vi "Real_Time_Main_Final_Digital.vi"() -> ()   [LabVIEW 2024]
uses:
  <vilib>/Platform/TimedLoop/XDataNode/timing_clust.ctl
  <vilib>/Platform/TimedLoop/XDataNode/nitl_modes.ctl
  <vilib>/Platform/TimedLoop/XDataNode/wakeup.ctl
  <instrlib>/niScope/Controls/niScope vertical coupling.ctl
  <instrlib>/niScope/Configure/Trigger/niScope Configure Trigger Digital.vi
  <instrlib>/niScope/Acquire/Fetch/niScope Fetch WDT.vi
  <vilib>/platform/TimedLoop/XDataNode/XDataNode.xnode
  <instrlib>/niScope/Controls/niScope trigger source digital.ctl
  <vilib>/Platform/TimedLoop/XDataNode/XDNodeRunTimeDep.lvlib
panel:
  out "output waveform":waveform(dbl)(graph)
  in  "trigger source":T1="VAL_RTSI_0"
  out "error out":errorcluster
  in  "Fetch:Fetch Relative To":i32(ring)=482 items=["Start"=482, "Trigger"=483, "Pretrigger"=477, "Now"=481, "Read Pointer"=388]
  out "# of Chunks Fetched":i32
  out "# of Points Fetched":i32
  out "Horizontal:Actual Sample Rate":dbl
  in  "channels":string="0"
  in  "stop":bool
  in  "Resource Name":refnum<k15>="Dev1" caption="Resource Name(s)"
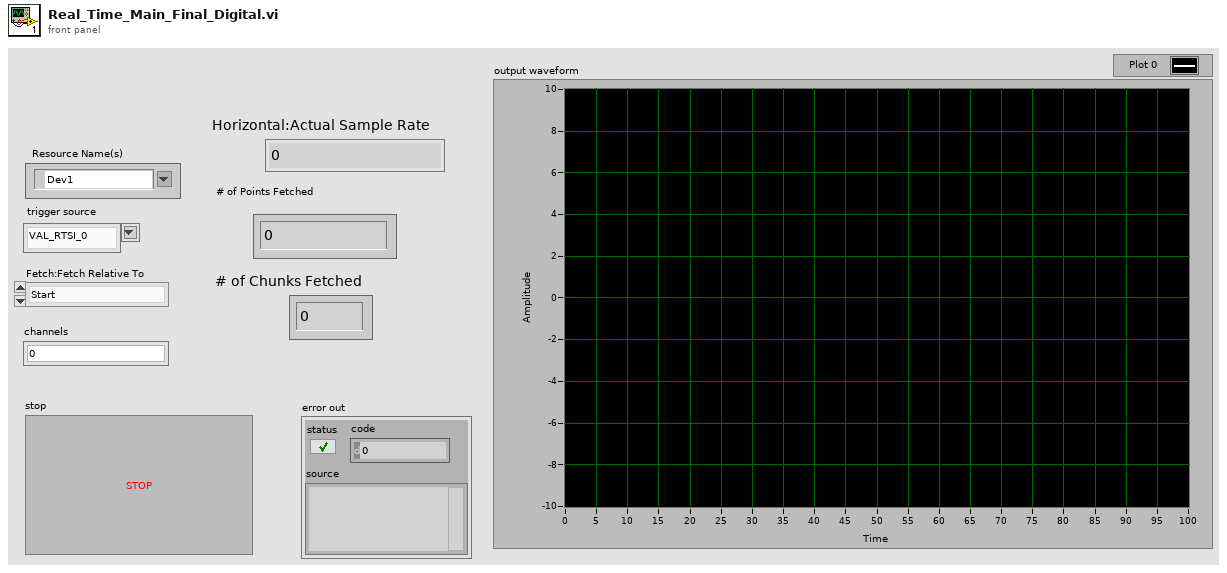
[diagram p1: front panel]
types:
  T1 = typedef "niScope trigger source digital.ctl" = string
  T2 = typedef "XDNodeRunTimeDep.lvlib/timing_clust.ctl" = cluster{"Expected End [f-1]":u64, "Actual End [f-1]":u64, "Finished Late? [f-1]":bool, "Expected End [i-1]":u64, "Actual End [i-1]":u64, "Finished Late? [i-1]":bool, "Expected Start [i]":u64, "Actual Start [i]":u64, "Expected Start [f]":u64, "Actual Start [f]":u64, "Source Name":string, "Structure Name":string, "Period":i64, "Deadline":i64, "Offset":i64, "Start":i64, "Priority":i32, "Timeout":i32, "Mode":T3, "Wakeup Reason":T4, "Error":errorcluster, "Source Type":string, "Secondary Source Type":string, "Global End Time":u64, "Global Start Time":u64, "Frame Duration":u64, "Iteration Duration":u64, "Assigned CPU":i32, "I/O Scan Engine Mode":u32}
  T3 = typedef "XDNodeRunTimeDep.lvlib/nitl_modes.ctl" = enum32{"No Change", "Process missed periods, maintain original phase", "Discard missed periods, maintain original phase", "Process missed periods, ignore original phase", "Discard missed periods, ignore original phase"}
  T4 = typedef "XDNodeRunTimeDep.lvlib/wakeup.ctl" = enum32{"Normal", "Aborted", "Asynchronous wakeup", "Timing source error", "Timed loop error", "Timeout"}
  T5 = typedef "niScope vertical coupling.ctl" = i32
  T6 = cluster{"actualSamples":i32, "absoluteInitialX":dbl, "relativeInitialX":dbl, "xIncrement":dbl, "offset":dbl, "gain":dbl, "reserved1":dbl, "reserved2":dbl}
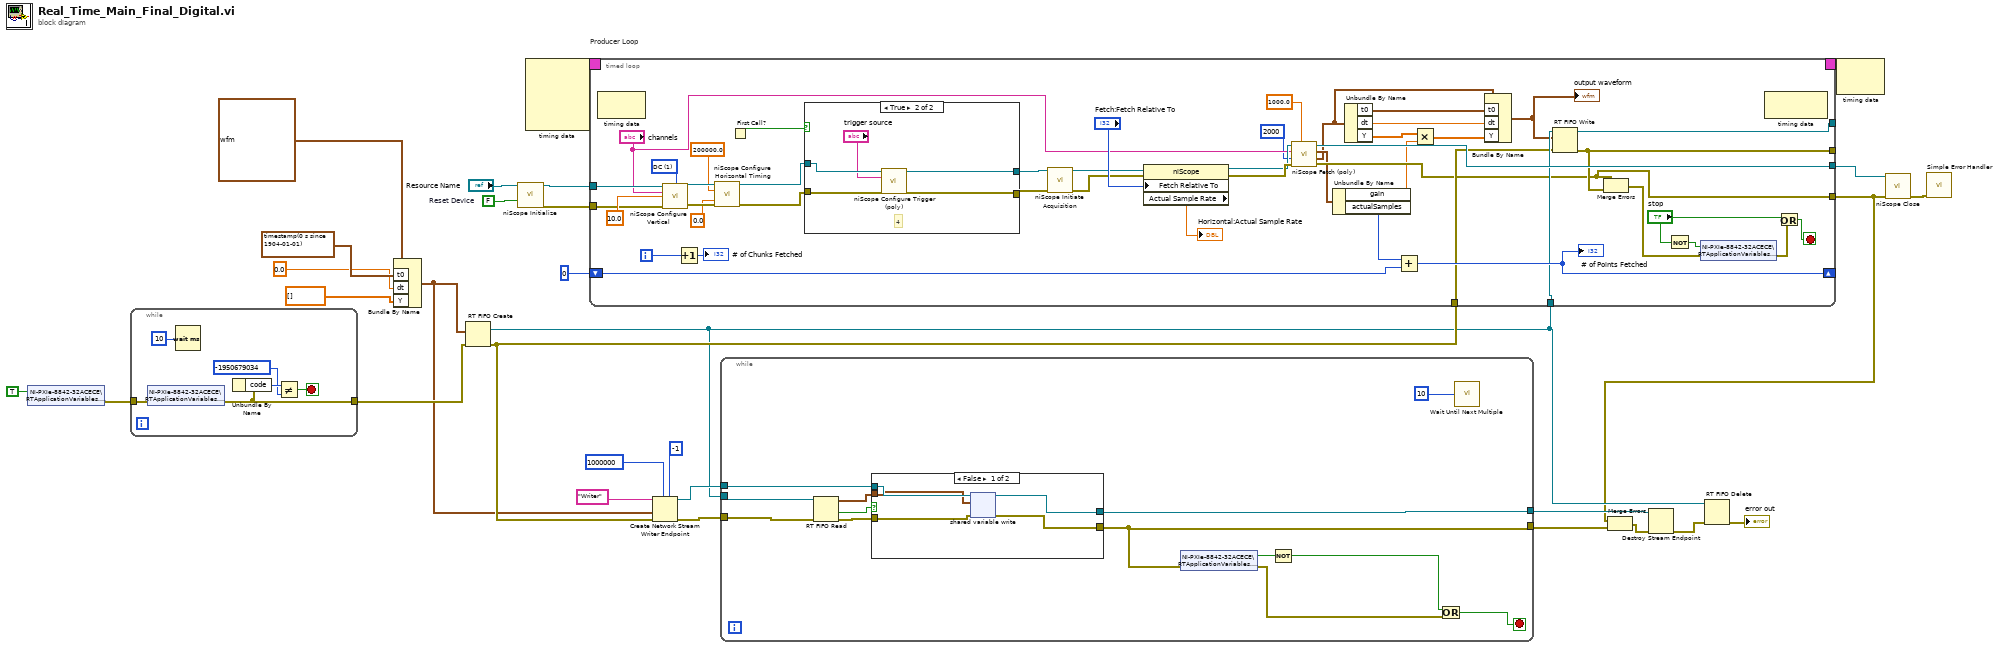
[diagram p0: block diagram]
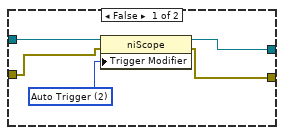
[diagram p3: hidden frame]
diagram:
  w28 = FALSE  # Reset Device
  n1 = shared-variable "NI-PXIe-8842-32ACECE\\RTApplicationVariables.lvlib\\Running?"(TRUE) -> (error out=w9:errorcluster)  [unwired: 1 in]
  n2 = while {
    tunnel: w9 -> [w36]
    tunnel: [w31] -> w8
    stop <- w33 stop-if-true
    n3 = shared-variable "NI-PXIe-8842-32ACECE\\RTApplicationVariables.lvlib\\Running?"(error in=w36) -> (error out=w31:errorcluster)  [unwired: 1 out]
    n4 = Wait (ms)(milliseconds to wait=u32 10) -> ()  [unwired: 1 out]
    n5 = Unbundle By Name(w31) -> ("code"=w35:i32)
    n6 = Not Equal?(x=w35, y=-1950679034) -> (x != y?=w33:bool)
  }
  n7 = Bundle By Name(cluster=waveform(dbl) {"t0"=timestamp(0 s since 1904-01-01), "dt"=1.0, "Y"=[]} ("waveform"), "t0"=timestamp(0 s since 1904-01-01), "dt"=0.0, "Y"=dbl[] []) -> (w3:waveform(dbl))
  n8 = RT FIFO Create(1:w3, 3:w8) -> (8:w11:refnum<k33>, 11:w21:errorcluster)  [unwired: 6 in, 1 out]
  n9 = call <instrlib>:"niScope Initialize.vi"("resource name"="Resource Name", "reset device"=w28) -> ("instrument handle"=w24:refnum<k15>, "error out"=w1:errorcluster)  [unwired: 12 in]
  n10 = node-c288() -> (w30:T2)  [unwired: 4 in]
  n11 = timed-loop "Producer Loop" {
    timing: w30 -> [_]
    timing-out: [_] -> w29
    tunnel: [w71] -> w26
    shift-right: [w69] -> _
    shift-left: 0 -> [w70]
    tunnel: w24 -> [w60]
    tunnel: w11 -> [w56]
    tunnel: w21 -> [w55]
    tunnel: [w54] -> _
    tunnel: [w53] -> _
    tunnel: [w47] -> w7
    tunnel: w1 -> [w37]
    i -> [w68]
    stop <- w50 stop-if-true
    w64 = T5 1 items=["AC", "DC", "Ground"] ("vertical coupling")
    n12 = node-c288() -> ()  [unwired: 1 in, 1 out]
    n13 = call <instrlib>:"niScope Configure Vertical.vi"("instrument handle"=w60, "vertical coupling"=w64, "channels"="channels", "vertical range"=10.0, "error in"=w37) -> ("instrument handle out"=w67:refnum<k15>, "error out"=w61:errorcluster)  [unwired: 9 in]
    n14 = Increment(x=w68) -> (x+1=→"# of Chunks Fetched":i32)
    n15 = call <instrlib>:"niScope Configure Horizontal Timing.vi"("instrument handle"=w67, "min sample rate"=200000.0, "reference position"=0.0, "error in"=w61) -> ("instrument handle out"=w62:refnum<k15>, "error out"=w63:errorcluster)  [unwired: 10 in]
    n16 = First Call?() -> (First Call?: T/F=w81:bool)
    n17 = case shown="True" w81 {
      tunnel: [w86 w92] -> w82
      tunnel: [w87 w91] -> w73
      tunnel: w63 -> [w84 w90]
      tunnel: w62 -> [w83 w89]
      frame False {
        w85 = 2 items=["None"=1, "Auto Trigger"=2] ("Triggering:Trigger Modifier")
        n18 = property class="niScope"(reference=w83, error in=w84, "Trigger Modifier"=w85) -> (reference out=w87:refnum<k15>, error out=w86:errorcluster)
      }
      frame True {
        # "4"
        n19 = call-poly <instrlib>:"niScope Configure Trigger (poly).vi"("instrument handle"=w89, "trigger source"="trigger source", "error in"=w90) -> ("instrument handle out"=w91:refnum<k15>, "error out"=w92:errorcluster)  [unwired: 11 in]
      }
    }
    n20 = call <instrlib>:"niScope Initiate Acquisition.vi"("instrument handle"=w73, "error in"=w82) -> ("instrument handle out"=w74:refnum<k15>, "error out"=w79:errorcluster)  [unwired: 12 in]
    n21 = property class="niScope"(reference=w74, error in=w79, "Fetch Relative To"="Fetch:Fetch Relative To") -> (reference out=w75:refnum<k15>, error out=w76:errorcluster, "Actual Sample Rate"=→"Horizontal:Actual Sample Rate":dbl)
    n22 = call-poly <instrlib>:"niScope Fetch (poly).vi"("timeout"=1000.0, "error in"=w76, "numSamples"=2000, "channels"="channels", "instrument handle"=w75) -> ("error out"=w47:errorcluster, "wfm"=w43:waveform(dbl), "wfm info"=w46:T6, "instrument handle out"=w71:refnum<k15>)  [unwired: 3 in]
    n23 = Unbundle By Name(w46) -> ("gain"=w40:dbl, "actualSamples"=w78:i32)
    n24 = Unbundle By Name(w43) -> ("t0"=w45:timestamp, "dt"=w44:dbl, "Y"=w42:dbl[])
    n25 = Add(x=w78, y=w70) -> (x+y=w69:i32)
    "# of Points Fetched" <- w69
    n26 = Multiply(x=w42, y=w40) -> (x*y=w41:dbl[])
    n27 = Bundle By Name(cluster=w43, "t0"=w45, "dt"=w44, "Y"=w41) -> (w38:waveform(dbl))
    "output waveform" <- w38
    n28 = RT FIFO Write(0:w56, 1:w38, 3:w55) -> (8:w54:refnum<k33>, 11:w53:errorcluster)  [unwired: 2 in, 2 out]
    n29 = Merge Errors(w47, w53) -> (w52:errorcluster)
    n30 = Not(x="stop") -> (.not. x?=w48:bool)
    n31 = shared-variable "NI-PXIe-8842-32ACECE\\RTApplicationVariables.lvlib\\Running?"(w48, error in=w52) -> (error out=w51:errorcluster)
    n32 = node-c288() -> ()  [unwired: 1 in, 1 out]
    n33 = Or(x="stop", y=w51) -> (x .or. y?=w50:bool)
  }
  n34 = Create Network Stream Writer Endpoint(5:-1 ("timeout in ms (-1)"), 7:1000000 ("writer buffer size"), 8:w21, 9:w3, 11:"Writer" ("writer name")) -> (0:w20:errorcluster, 3:w19:refnum<k21>)  [unwired: 2 in]
  n35 = while {
    tunnel: w20 -> [w107]
    tunnel: w11 -> [w104]
    tunnel: w19 -> [w102]
    tunnel: [w98] -> w14
    tunnel: [w100] -> w13
    stop <- w95 stop-if-true
    n36 = RT FIFO Read(0:w104, 3:w107) -> (9:w105:waveform(dbl), 10:w106:bool, 11:w103:errorcluster)  [unwired: 2 in, 2 out]
    n37 = case shown="False" w106 {
      tunnel: w105 -> [w108 _]
      tunnel: w103 -> [w109 w113]
      tunnel: w102 -> [w110 w114]
      tunnel: [w111 w113] -> w98
      tunnel: [w112 w114] -> w100
      frame False {
        n38 = shared-variable-write(w110, w109, w108) -> (w112:refnum<k21>, w111:errorcluster)  [unwired: 1 in, 1 out]
      }
      frame True {
      }
    }
    n39 = shared-variable "NI-PXIe-8842-32ACECE\\RTApplicationVariables.lvlib\\Running?"(error in=w98) -> (w99:bool, error out=w96:errorcluster)
    n40 = Not(x=w99) -> (.not. x?=w97:bool)
    n41 = Or(x=w97, y=w96) -> (x .or. y?=w95:bool)
    n42 = call "Wait Until Next Multiple"("Count(mSec)"=u32 10) -> ()  [unwired: 1 out]
  }
  n43 = Merge Errors(w7, w14) -> (w17:errorcluster)
  n44 = Destroy Stream Endpoint(8:w17, 11:w13) -> (0:w18:errorcluster)
  n45 = RT FIFO Delete(0:w11, 3:w18) -> (11:→"error out":errorcluster)  [unwired: 1 in]
  n46 = node-c288(w29) -> ()  [unwired: 1 out]
  n47 = call <instrlib>:"niScope Close.vi"("instrument handle"=w26, "error in"=w7) -> ("error out"=w15:errorcluster)  [unwired: 13 in]
  n48 = call <vilib>:"Simple Error Handler.vi"("error in (no error)"=w15) -> ()  [unwired: 4 in, 5 out]
